vi "ZBX Set Gain.vi"(7 "channel":T1, 8 "response":T2, 9 "input valid":bool=TRUE, 10 "config index":u32, 11 "gain":u32) -> (0 "ready for input":bool=TRUE, 3 "request":T3)   [LabVIEW 2023]
doc: "Change gain value for the selected DBoardState (config index) and RF path. The gain value will be applied immediately. \nNote: The gain change will have immediate effect if the current DBoardState is active. Otherwise it will get active when the DBoardState changes to the given state."
uses:
  <instrlib>/niUSRP/Reference FPGA/ZBX Control/ZBX IO Request.ctl
  <instrlib>/niUSRP/Reference FPGA/ZBX Control/ZBX IO Response.ctl
  <instrlib>/niUSRP/Reference FPGA/ZBX Control/Antenna.ctl
panel:
  out "result":u32
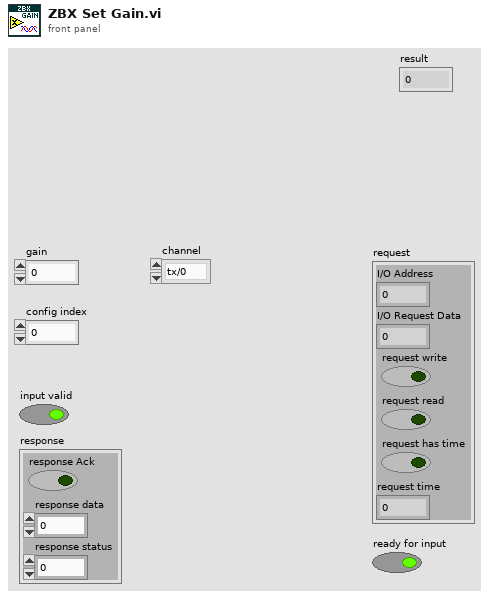
[diagram p1: front panel]
types:
  T1 = typedef "Antenna.ctl" = enum8{"tx/0", "tx/1", "rx/0", "rx/1"}
  T2 = typedef "ZBX IO Response.ctl" = cluster{"response Ack":bool, "response data":u32, "response status":fxp<+,2,2>}
  T3 = typedef "ZBX IO Request.ctl" = cluster{"I/O Address":fxp<+,20,20>, "I/O Request Data":u32, "request write":bool, "request read":bool, "request has time":bool, "request time":u64}
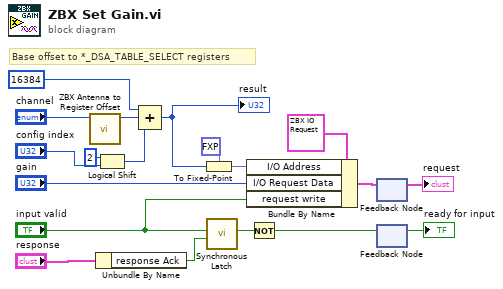
[diagram p0: block diagram]
diagram:
  # "Base offset to *_DSA_TABLE_SELECT registers"
  n1 = call <instrlib>:"ZBX Antenna to Register Offset.vi"("Antenna"="channel") -> ("register offset"=w11:u32)  [unwired: 10 in]
  n2 = Unbundle By Name("response") -> ("response Ack"=w16:bool)
  n3 = Logical Shift(y=i16 2, x="config index") -> (x << y=w7:u32)
  n4 = Compound Arithmetic op=ADD(u32 16384 ("config index"), w11, w7) -> (w10:u32)
  "result" <- w10
  n5 = To Fixed-Point(fixed-point type=fxp<+,20,20> 0.0 ("I/O Address"), number=w10) -> (fixed-point=w5:fxp<+,20,20>)
  n6 = call <instrlib>:"Synchronous Latch.vi"("clear"=w16, "set"="input valid") -> ("out"=w17:bool)  [unwired: 9 in]
  n7 = Bundle By Name(cluster=T3 {"I/O Address"=0.0, "I/O Request Data"=0, "request write"=FALSE, "request read"=FALSE, "request has time"=FALSE, "request time"=0} ("request"), "I/O Address"=w5, "I/O Request Data"="gain", "request write"="input valid") -> (w2:T3)
  n8 = Not(x=w17) -> (.not. x?=w4:bool)
  n9 = feedback-in #1(w2) -> ()
  n10 = feedback #1() -> (→"request":T3)  [unwired: 1 in]
  n11 = feedback #2() -> (→"ready for input":bool)  [unwired: 1 in]
  n12 = feedback-in #2(w4) -> ()
